vi "Pixy SPI.vi"() -> ()   [LabVIEW 2016]
doc: "This example shows how to communicate and interpret data for a PIXY camera."
uses:
  <vilib>/Rock Robotics/SystemInterfaces/spilib/spi_bus.ctl
  <vilib>/Rock Robotics/WPI/SPI/WPI_SPIMode.ctl
panel:
  in  "SPI Bus":T1=enum."Invalid"
  in  "CC Objects":bool=TRUE
  in  "Objects":bool=TRUE
  out "CC Objects":T2(array[cluster])
  out "Totals":T3
  in  "Image Brightness":u8(slide)=80 scale=0.0..255.0
  out "ms between frames":u32(graph)
  in  "Shape Colors":u32[](array[colorbox])=[16748288, 16746709, 1244948]
  in  "LED Color":cluster{"Red":u8, "Green":u8, "Blue":u8} {"Blue" scale=0.0..255.0; "Green" scale=0.0..255.0; "Red" scale=0.0..255.0}
  out "Picture":picture
  out "Objects":T4(array[cluster])
  # "SPI cable\nPin 1 -> MISO\nPin 3 -> SCK\nPin 4 -> MOSI\nPin 7 -> CS(0, 1, 2, or 3)\nPin 10 -> GND"
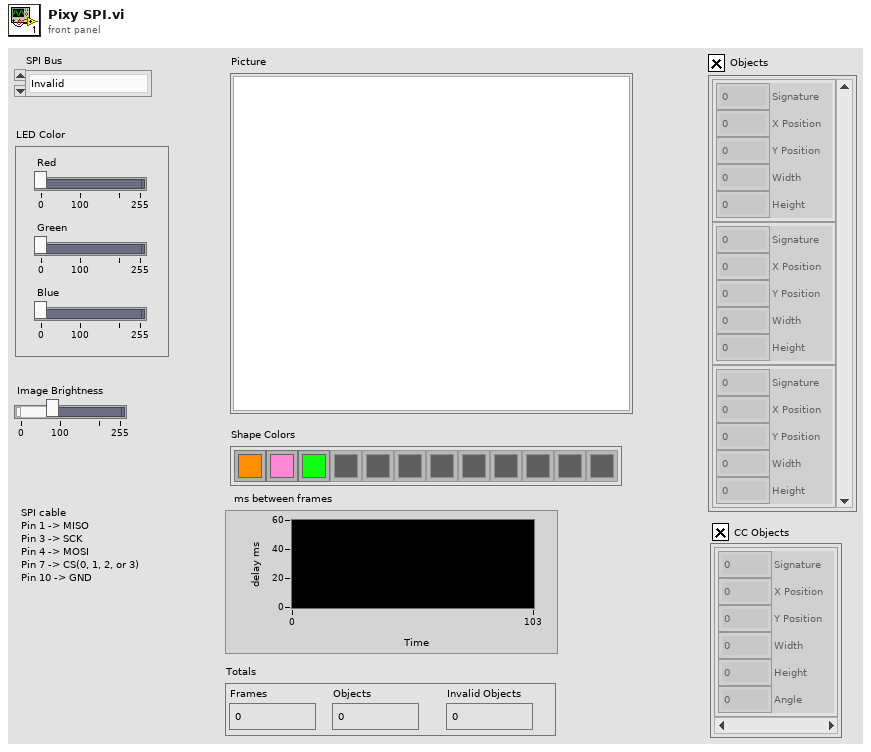
[diagram p1: front panel]
types:
  T1 = typedef "spi_bus.ctl" = enum16{"SPI On-Board, CS0", "SPI On-Board, CS1", "SPI On-Board, CS2", "SPI On-Board, CS3", "SPI MXP", "Invalid"}
  T2 = cluster{"Signature":u16, "X Position":u16, "Y Position":u16, "Width":u16, "Height":u16, "Angle":i16}[]
  T3 = cluster{"Frames":u32, "Objects":u32, "Invalid Objects":i32}
  T4 = cluster{"Signature":u16, "X Position":u16, "Y Position":u16, "Width":u16, "Height":u16}[]
  T5 = typedef "WPI_SPIMode.ctl" = enum16{"Mode 0 (Clk Idle Low,Sample on Leading)", "Mode 1 (Clk Idle Low,Sample on Trailing)", "Mode 2 (Clk Idle High,Sample on Leading)", "Mode 3 (Clk Idle High,Sample on Trailing)"}
  T6 = enum16{"Read Objects", "Write LED Color", "Write Brightness", "Write Objects", "Read Settings"}
  T7 = typedef "WPI_SPIDevRef.ctl" = cluster{"DevStatus":errorcluster, "Handle":i32, "SPI Bus":T1}
  T8 = cluster{"Signature":u16, "X Position":u16, "Y Position":u16, "Width":u16, "Height":u16}
  T9 = cluster{"Signature":u16, "X Position":u16, "Y Position":u16, "Width":u16, "Height":u16, "Angle":i16}
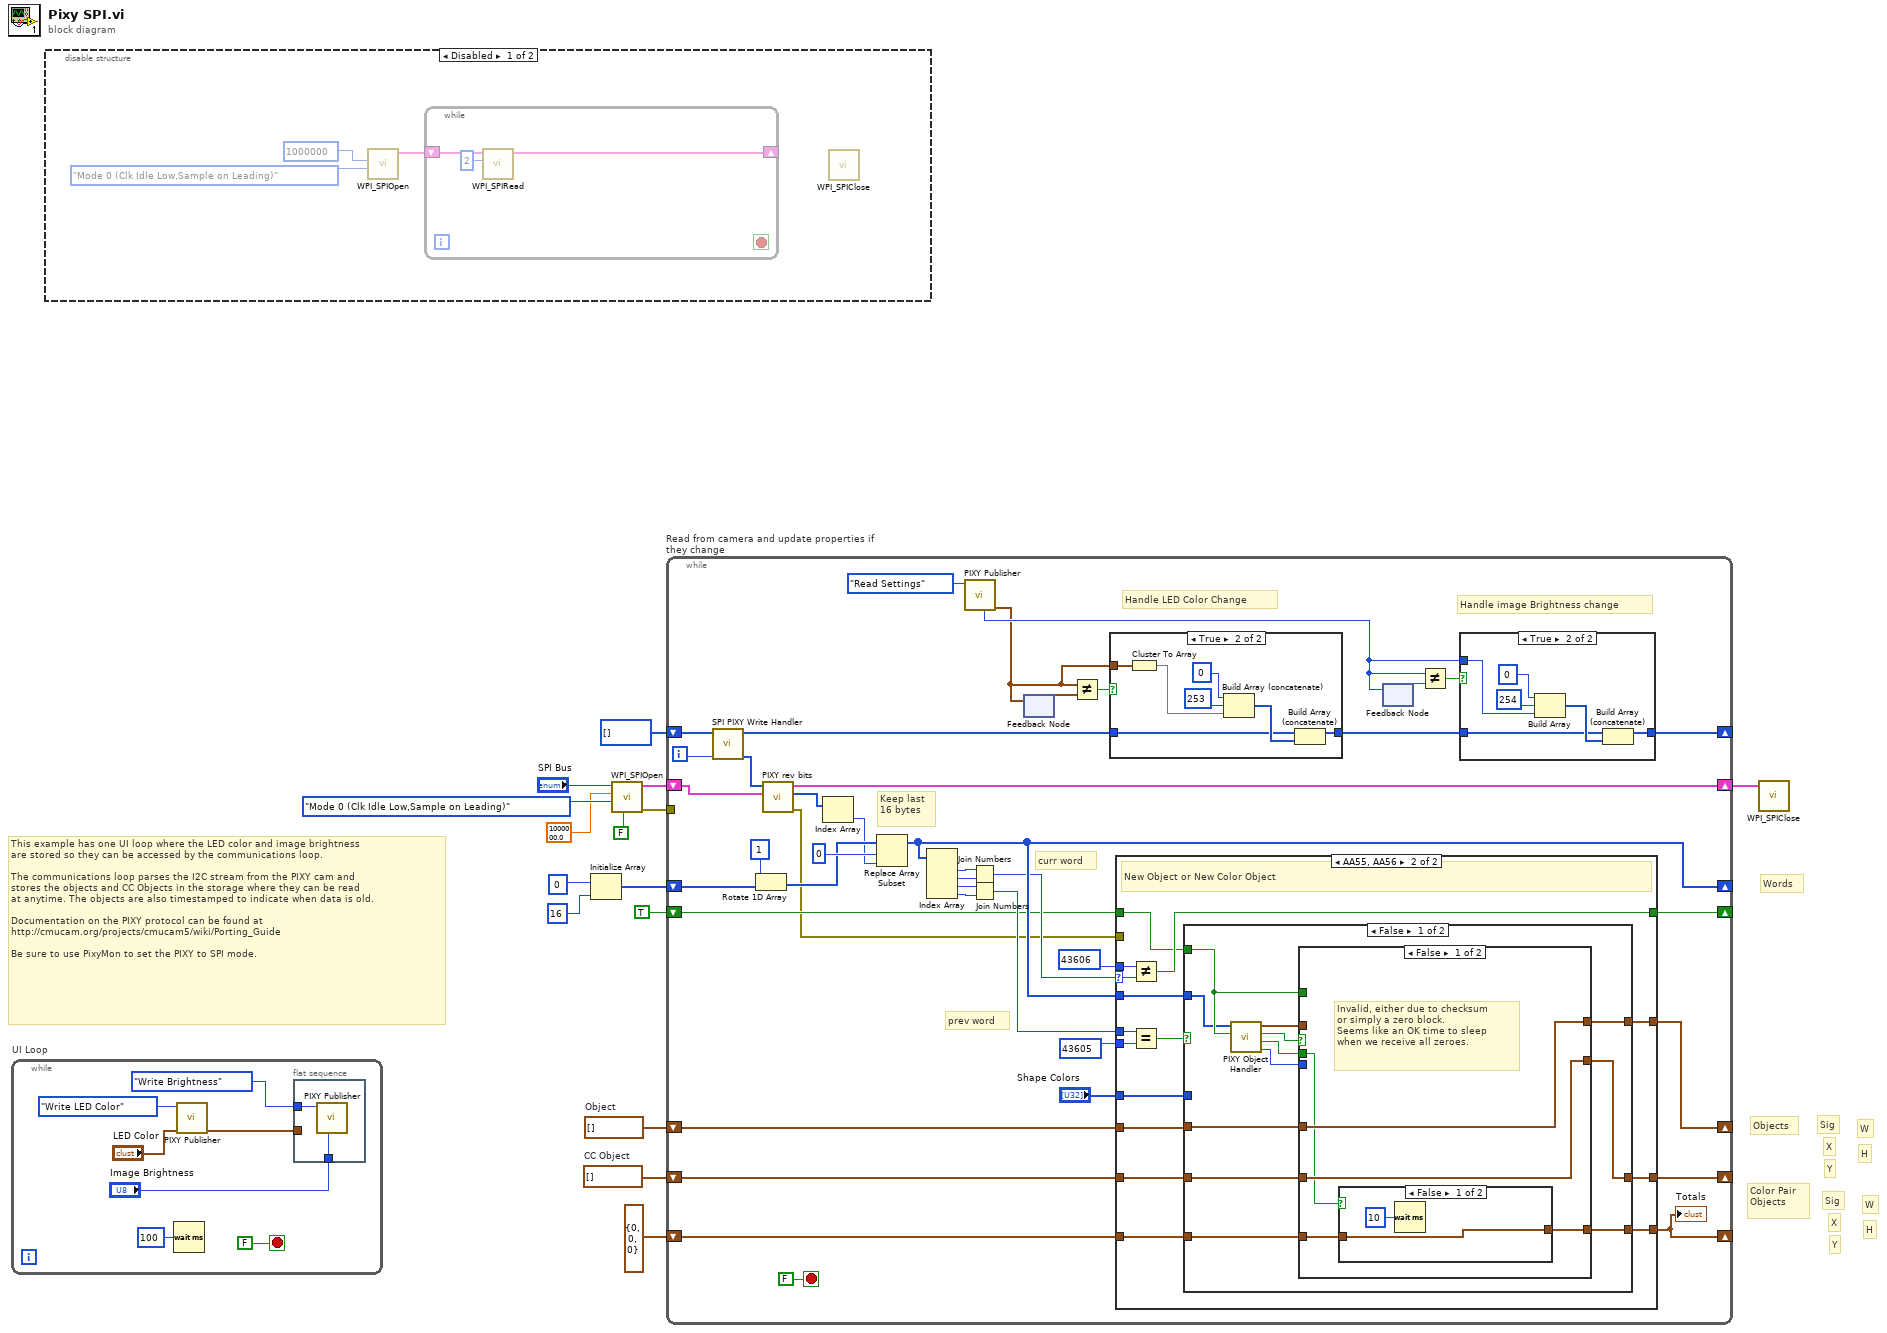
[diagram p0: block diagram]
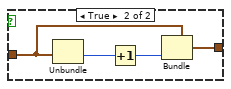
[diagram p3: hidden frame]
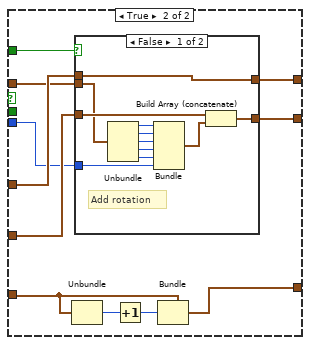
[diagram p4: hidden frame]
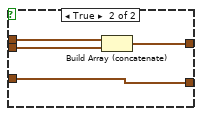
[diagram p5: hidden frame]
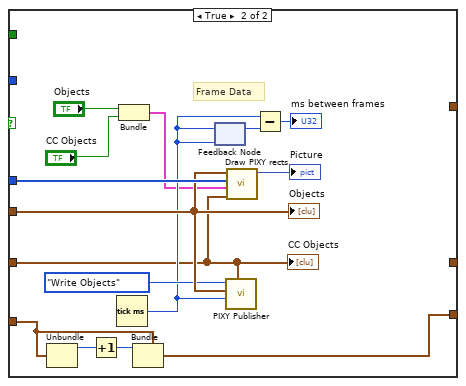
[diagram p6: hidden frame]
diagram:
  w11 = T2 []  # CC Object
  w12 = T4 []  # Object
  # "This example has one UI loop where the LED color and image brightness\nare stored so they can be accessed by the communications loop.\n\nThe communications loop parses the I2C stream from the PIXY cam and\nstores the objects and CC Objects in the storage where they can be read\nat anytime. The objects are also timestamped to indicate when data is old.\n\nDocumentation on the PIXY protocol can be found at\nhttp://cmucam.org/projects/cmucam5/wiki/Porting_Guide\n\nBe sure to use PixyMon to set the PIXY to SPI mode."
  # "H"
  # "W"
  # "Y"
  # "X"
  # "Sig"
  # "Color Pair\nObjects"
  # "H"
  # "W"
  # "Y"
  # "X"
  # "Sig"
  # "Objects"
  # "Words"
  n1 = while "UI Loop" {
    stop <- FALSE stop-if-true
    n2 = Wait (ms)(milliseconds to wait=u32 100) -> ()  [unwired: 1 out]
    n3 = call "PIXY Publisher.vi"("Color"="LED Color", "Operation"=T6."Write LED Color") -> ("Color Out"=w17:cluster{"Red":u8, "Green":u8, "Blue":u8})  [unwired: 5 in, 4 out]
    n4 = flat-sequence {
      tunnel: T6."Write Brightness" ("Operation") -> [w24]
      tunnel: "Image Brightness" -> [w23]
      tunnel: w17 -> [_]
      frame #0 {
        n5 = call "PIXY Publisher.vi"("Brightness"=w23, "Operation"=w24) -> ()  [unwired: 5 in, 5 out]
      }
    }
  }
  n6 = disable-structure shown="Disabled" {
    frame Disabled {
      n7 = call <vilib>:"WPI_SPIOpen.vi"("Mode (3)"=WPI_SPIMode."Mode 0 (Clk Idle Low,Sample on Leading)", "Clock Rate (Hz)"=1000000) -> ("SPIDevRef"=w25:T7)  [unwired: 4 in, 5 out]
      n8 = while {
        shift-right: [w28] -> _
        shift-left: w25 -> [w30]
        stop <- _ stop-if-true
        n9 = call <vilib>:"WPI_SPIRead.vi"("Num to Read"=2, "SPIDevRef"=w30) -> ("SPIDevRef"=w28:T7)  [unwired: 7 in, 2 out]
      }
      n10 = call <vilib>:"WPI_SPIClose.vi"() -> ()  [unwired: 11 in, 1 out]
    }
    frame Enabled {
    }
  }
  n11 = Initialize Array(u8 0 ("Num to Read"), 16 ("Num to Read")) -> (w13:u8[])
  n12 = call <vilib>:"WPI_SPIOpen.vi"("Chip Select Active High (F)"=FALSE, "Mode (3)"=WPI_SPIMode."Mode 0 (Clk Idle Low,Sample on Leading)", "Clock Rate (Hz)"=1000000.0, "SPI Bus"="SPI Bus") -> ("error out"=w4:errorcluster, "SPIDevRef"=w7:T7)  [unwired: 6 in]
  n13 = while "Read from camera and update properties if they change" {
    shift-right: [w36] -> w3
    shift-left: w7 -> [w39]
    shift-right: [w46] -> _
    shift-left: w13 -> [w65]
    shift-right: [w67] -> _
    shift-left: w12 -> [w68]
    shift-right: [w60] -> _
    shift-left: w11 -> [w61]
    shift-right: [w42] -> _
    shift-left: T3 {"Frames"=0, "Objects"=0, "Invalid Objects"=0} ("Totals") -> [w43]
    shift-right: [w40] -> _
    shift-left: TRUE -> [w41]
    tunnel: w4 -> [_]
    shift-right: [w35] -> _
    shift-left: u8[] [] -> [w33]
    i -> [w31]
    stop <- FALSE stop-if-true
    # "curr word"
    # "Handle image Brightness change"
    # "Handle LED Color Change"
    # "prev word"
    # "Keep last\n16 bytes"
    n14 = call "SPI PIXY Write Handler.vi"("index"=w31, "Write Buffer"=w33) -> ("SPI to Send"=w32:u8[], "Write Buffer out"=w34:u8[])  [unwired: 8 in]
    n15 = Rotate 1D Array(1:w65, 2:1 ("Num to Read")) -> (0:w66:u8[])
    n16 = call "PIXY rev bits.vi"("SPIDevRef in"=w39, "SPI to Send"=w32) -> ("error out"=w38:errorcluster, "Received Data"=w37:u8[], "SPIDevRef out"=w36:T7)  [unwired: 7 in]
    n17 = Index Array(array=w37) -> (element=w52:u8)  [unwired: 1 in]
    n18 = Replace Array Subset(array=w66, new element=w52, index=0 ("Num to Read")) -> (w46:u8[])
    n19 = Index Array(array=w46) -> (element #1=w51:u8, element #2=w50:u8, element #3=w49:u8, element #4=w48:u8)  [unwired: 4 in]
    n20 = call "PIXY Publisher.vi"("Operation"=T6."Read Settings") -> ("Color Out"=w57:cluster{"Red":u8, "Green":u8, "Blue":u8}, "Brightness Out"=w58:u8)  [unwired: 6 in, 3 out]
    n21 = Join Numbers(hi=w51, lo=w50) -> ((hi.lo)=w45:u16)
    n22 = Join Numbers(hi=w49, lo=w48) -> ((hi.lo)=w47:u16)
    n23 = feedback #1() -> (w64:cluster{"Red":u8, "Green":u8, "Blue":u8})  [unwired: 1 in]
    n24 = feedback-in #1(w57) -> ()
    n25 = Not Equal?(x=w57, y=w64) -> (x != y?=w63:bool)
    n26 = case shown="True" w63 {
      tunnel: w34 -> [w162 w164]
      tunnel: [w162 w163] -> w62
      tunnel: w57 -> [_ w169]
      frame False {
      }
      frame True {
        n27 = Cluster To Array(cluster=w169) -> (array=w168:u8[])
        n28 = Build Array (concatenate)(u8 0 ("Num to Read"), u8 253 ("Num to Read"), w168) -> (w165:u8[])
        n29 = Build Array (concatenate)(w164, w165) -> (w163:u8[])
      }
    }
    n30 = case shown="AA55, AA56" w45 {
      selector: w45 -> [_ w85]
      tunnel: w47 -> [_ w90]
      tunnel: u16 43605 ("Num to Read") -> [_ w89]
      tunnel: w68 -> [w75 w88]
      tunnel: [w75 w87] -> w67
      tunnel: w46 -> [_ w81]
      tunnel: u16 43606 ("Num to Read") -> [_ w84]
      tunnel: w61 -> [w74 w83]
      tunnel: [w74 w82] -> w60
      tunnel: w38 -> [_ _]
      tunnel: "Shape Colors" -> [_ w80]
      tunnel: w43 -> [w73 w79]
      tunnel: [w73 w78] -> w42
      tunnel: w41 -> [w72 w76]
      tunnel: [w72 w77] -> w40
      frame Default {
        # "Nothing to do, already appended"
        # "Just another word for the object"
      }
      frame 43605, 43606 {
        # "New Object or New Color Object"
        n31 = Not Equal?(x=w84, y=w85) -> (x != y?=w77:bool)
        n32 = Equal?(x=w90, y=w89) -> (x = y?=w86:bool)
        n33 = case shown="False" w86 {
          tunnel: w88 -> [w102 w150]
          tunnel: [w101 _] -> w87
          tunnel: w80 -> [_ w152]
          tunnel: w83 -> [w100 w143]
          tunnel: w76 -> [w95 _]
          tunnel: [w99 _] -> w82
          tunnel: w81 -> [w93 _]
          tunnel: w79 -> [w92 w147]
          tunnel: [w91 w146] -> w78
          frame False {
            n34 = call "PIXY Object Handler.vi"("Normal Object"=w95, "Accumulated Words"=w93) -> ("Angle"=w94:i16, "CheckSum Error"=w96:bool, "Valid"=w97:bool, "Object"=w98:T8)  [unwired: 6 in]
            n35 = case shown="False" w97 {
              tunnel: w102 -> [w107 w124]
              tunnel: [w107 w123] -> w101
              tunnel: w100 -> [w106 w122]
              tunnel: w95 -> [_ w121]
              tunnel: [w106 w120] -> w99
              tunnel: w98 -> [_ w119]
              tunnel: w96 -> [w105 _]
              tunnel: w94 -> [_ w118]
              tunnel: w92 -> [w104 w117]
              tunnel: [w103 w116] -> w91
              frame False {
                # "Invalid, either due to checksum\nor simply a zero block.\nSeems like an OK time to sleep\nwhen we receive all zeroes."
                n36 = case shown="False" w105 {
                  tunnel: w104 -> [w109 w111]
                  tunnel: [w109 w113] -> w103
                  frame False {
                    n37 = Wait (ms)(milliseconds to wait=u32 10) -> ()  [unwired: 1 out]
                  }
                  frame True {
                    n38 = Unbundle(w111) -> ("Invalid Objects"=w112:i32)  [unwired: 2 out]
                    n39 = Increment(x=w112) -> (x+1=w110:i32)
                    n40 = Bundle(cluster=w111, "Invalid Objects"=w110) -> (w113:T3)  [unwired: 2 in]
                  }
                }
              }
              frame True {
                n41 = Unbundle(w117) -> ("Objects"=w115:u32)  [unwired: 2 out]
                n42 = case shown="False" w121 {
                  tunnel: w119 -> [w129 w139]
                  tunnel: w124 -> [w135 w138]
                  tunnel: [w135 w137] -> w123
                  tunnel: w122 -> [w134 w136]
                  tunnel: [w133 w136] -> w120
                  tunnel: w118 -> [w125 _]
                  frame False {
                    # "Add rotation"
                    n43 = Unbundle(w129) -> ("Signature"=w131:u16, "X Position"=w130:u16, "Y Position"=w128:u16, "Width"=w127:u16, "Height"=w126:u16)
                    n44 = Bundle("Signature"=w131, "X Position"=w130, "Y Position"=w128, "Width"=w127, "Height"=w126, "Angle"=w125) -> (w132:T9)  [unwired: 1 in]
                    n45 = Build Array (concatenate)(w134, w132) -> (w133:T2)
                  }
                  frame True {
                    n46 = Build Array (concatenate)(w138, w139) -> (w137:T4)
                  }
                }
                n47 = Increment(x=w115) -> (x+1=w114:u32)
                n48 = Bundle(cluster=w117, "Objects"=w114) -> (w116:T3)  [unwired: 2 in]
              }
            }
          }
          frame True {
            # "Frame Data"
            n49 = Unbundle(w147) -> ("Frames"=w145:u32)  [unwired: 2 out]
            n50 = Increment(x=w145) -> (x+1=w144:u32)
            n51 = Tick Count (ms)() -> (millisecond timer value=w148:u32)
            n52 = Bundle("Objects"="Objects", "CC Objects"="CC Objects") -> (w142:cluster{"Objects":bool, "CC Objects":bool})  [unwired: 1 in]
            n53 = Bundle(cluster=w147, "Frames"=w144) -> (w146:T3)  [unwired: 2 in]
            n54 = feedback #2(w148) -> (w154:u32)
            n55 = feedback-in #2(w148) -> ()
            n56 = call "PIXY Publisher.vi"("Color Combo Object"=w143, "TimeStamp in"=w148, "Object"=w150, "Operation"=T6."Write Objects") -> ()  [unwired: 3 in, 5 out]
            n57 = call "Draw PIXY rects.vi"("CC Objects"=w143, "Draw Options"=w142, "Colors"=w152, "Object"=w150) -> ("Picture"=→"Picture":picture)  [unwired: 7 in]
            n58 = Subtract(x=w148, y=w154) -> (x-y=→"ms between frames":u32)
            "Objects" <- w150
            "CC Objects" <- w143
          }
        }
      }
    }
    "Totals" <- w42
    n59 = feedback #3() -> (w56:u8)  [unwired: 1 in]
    n60 = feedback-in #3(w58) -> ()
    n61 = Not Equal?(x=w58, y=w56) -> (x != y?=w55:bool)
    n62 = case shown="True" w55 {
      tunnel: w62 -> [w155 w157]
      tunnel: [w155 w156] -> w35
      tunnel: w58 -> [_ w160]
      frame False {
      }
      frame True {
        n63 = Build Array(u8 0 ("Num to Read"), u8 254 ("Num to Read"), w160) -> (w158:u8[])
        n64 = Build Array (concatenate)(w157, w158) -> (w156:u8[])
      }
    }
  }
  n65 = call <vilib>:"WPI_SPIClose.vi"("SPIDevRef"=w3) -> ()  [unwired: 10 in, 1 out]
